vi "5GNR_Example.vi"() -> ()   [LabVIEW 2016]
uses:
  Source/SA/RFmxNR/Typedefs/NR ModAcc Configuration.ctl
  Source/SA/RFmxNR/Typedefs/NR ModAcc Results.ctl
  Source/SA/RFmxNR/Typedefs/NR ModAcc Component Carrier Results.ctl
  Source/Common/SA Common Configuration.ctl
  Source/SA/RFmxNR/Typedefs/NR Standard Configuration.ctl
  Source/SA/RFmxInstr/Typedefs/Instrument Configuration.ctl
  Source/Common/Local Oscillator Sharing Mode.ctl
  Source/Common/SA Auto Level Configuration.ctl
  Source/SA/RFmxNR/RFmxNR.lvlib
  Source/SA/RFmxInstr/RFmxInstr.lvlib
  Source/Common/Common.lvlib
panel:
  out "error out":errorcluster
  out "ModAcc Results":T1
  in  "Tab Control":enum32{"Common", "Standard", "ModAcc"}(tab)=enum."ModAcc"
  in  "Resource Name":refnum<k15>="VST"
  in  "Common Configuration":T3={"Center Frequency (Hz)"=3500000000.0, "Reference Level (dBm)"=0.0, "External Attenuation (dB)"=0.0, "Trigger Enabled"=TRUE, "Digital Trigger Source"="PXI_Trig0", "Trigger Delay (s)"=0.0, "Selected Ports"=""} {"Trigger Delay (s)" format="%.2p"; "External Attenuation (dB)" format="%.2f"; "Reference Level (dBm)" format="%.2f"; "Center Frequency (Hz)" format="%.6p"}
  in  "Instrument Configuration":T4={"LO Sharing Mode"=enum."Automatic", "Frequency Reference Source"="PXI_Clk"}
  in  "Auto Level Configuration":T6={"Enabled"=TRUE, "Measurement Interval (s)"=0.01} {"Measurement Interval (s)" min=1e-06 max=100.0 format="%.2p"}
  in  "NR Standard Configuration":T7={"Link Direction"=1, "Frequency Range"=0, "Band"=78, "Auto Resource Block Detection Enabled"=1, "Downlink Test Model"=0, "Downlink Test Model Duplex Scheme"=0, "Component Carrier Configurations"=[{"Bandwidth (Hz)"=100000000.0, "Cell ID"=0, "PUSCH Modulation Type"=1, "Subcarrier Spacing (Hz)"=30000.0, "PUSCH Resource Block Offset"=0, "PUSCH Number of Resource Blocks"=-1, "PUSCH Transform Precoding Enabled"=0, "PUSCH Slot Allocation"="0-Last", "PUSCH Symbol Allocation"="0-Last", "PUSCH DMRS Configuration Type"=0, "PUSCH Mapping Type"=0, "PUSCH DMRS Type A Position"=2, "PUSCH DMRS Duration"=1, "PUSCH DMRS Additional Positions"=0}]} {"Downlink Test Model Duplex Scheme" items=["FDD", "TDD"]; "Downlink Test Model" items=["TM1.1", "TM1.2", "TM2", "TM2a", "TM3.1", "TM3.1a", "TM3.2", "TM3.3"]; "Component Carrier Configurations"."PUSCH DMRS Additional Positions" items=["0", "1", "2", "3"]; "Component Carrier Configurations"."PUSCH DMRS Duration" items=["Single-Symbol"=1, "Double-Symbol"=2]; "Component Carrier Configurations"."PUSCH DMRS Type A Position" items=["2"=2, "3"=3]; "Component Carrier Configurations"."PUSCH Mapping Type" items=["Type A", "Type B"]; "Component Carrier Configurations"."PUSCH DMRS Configuration Type" items=["Type 1", "Type 2"]; "Component Carrier Configurations"."PUSCH Transform Precoding Enabled" items=["False", "True"]; "Component Carrier Configurations"."Subcarrier Spacing (Hz)" items=["15kHz"=15000.0, "30kHz"=30000.0, "60kHz"=60000.0, "120kHz"=120000.0]; "Component Carrier Configurations"."PUSCH Modulation Type" items=["PI/2 BPSK", "QPSK", "16 QAM", "64 QAM", "256 QAM"]; "Component Carrier Configurations"."Bandwidth (Hz)" items=["5M"=5000000.0, "10M"=10000000.0, "15M"=15000000.0, "20M"=20000000.0, "25M"=25000000.0, "30M"=30000000.0, "40M"=40000000.0, "50M"=50000000.0, "60M"=60000000.0, "70M"=70000000.0, "80M"=80000000.0, "90M"=90000000.0, "100M"=100000000.0, "200M"=200000000.0, "400M"=400000000.0]; "Auto Resource Block Detection Enabled" items=["False", "True"]; "Frequency Range" items=["Range 1", "Range 2"]; "Link Direction" items=["Downlink", "Uplink"]}
  in  "ModAcc Configuration":T8={"Measurement Length Unit"=1, "Measurement Offset"=0.0, "Measurement Length"=1.0, "EVM Unit"=0, "Averaging Enabled"=0, "Averaging Count"=10} {"Averaging Enabled" items=["False", "True"]; "EVM Unit" items=["Percentage", "dB"]; "Measurement Length Unit" items=["Slot"=1, "Subframe"=3, "Time"=6]}
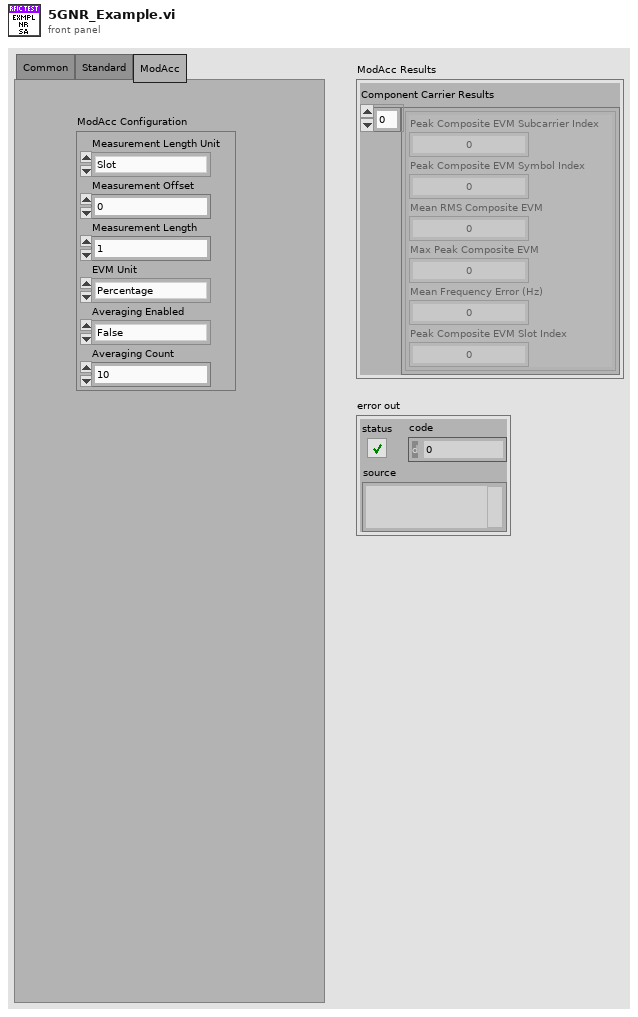
[diagram p1: front panel]
types:
  T1 = typedef "RFmxNR.lvlib/NR ModAcc Results.ctl" = cluster{"Component Carrier Results":T2[]}
  T2 = typedef "RFmxNR.lvlib/NR ModAcc Component Carrier Results.ctl" = cluster{"Peak Composite EVM Subcarrier Index":i32, "Peak Composite EVM Symbol Index":i32, "Mean RMS Composite EVM":dbl, "Max Peak Composite EVM":dbl, "Mean Frequency Error (Hz)":dbl, "Peak Composite EVM Slot Index":i32}
  T3 = typedef "Common.lvlib/SA Common Configuration.ctl" = cluster{"Center Frequency (Hz)":dbl, "Reference Level (dBm)":dbl, "External Attenuation (dB)":dbl, "Trigger Enabled":bool, "Digital Trigger Source":string, "Trigger Delay (s)":dbl, "Selected Ports":string}
  T4 = typedef "RFmxInstr.lvlib/Instrument Configuration.ctl" = cluster{"LO Sharing Mode":T5, "Frequency Reference Source":string}
  T5 = typedef "Common.lvlib/Local Oscillator Sharing Mode.ctl" = enum16{"Automatic", "None"}
  T6 = typedef "Common.lvlib/SA Auto Level Configuration.ctl" = cluster{"Enabled":bool, "Measurement Interval (s)":dbl}
  T7 = typedef "RFmxNR.lvlib/NR Standard Configuration.ctl" = cluster{"Link Direction":i32, "Frequency Range":i32, "Band":i32, "Auto Resource Block Detection Enabled":i32, "Downlink Test Model":i32, "Downlink Test Model Duplex Scheme":i32, "Component Carrier Configurations":cluster{"Bandwidth (Hz)":dbl, "Cell ID":i32, "PUSCH Modulation Type":i32, "Subcarrier Spacing (Hz)":dbl, "PUSCH Resource Block Offset":i32, "PUSCH Number of Resource Blocks":i32, "PUSCH Transform Precoding Enabled":i32, "PUSCH Slot Allocation":string, "PUSCH Symbol Allocation":string, "PUSCH DMRS Configuration Type":i32, "PUSCH Mapping Type":i32, "PUSCH DMRS Type A Position":i32, "PUSCH DMRS Duration":i32, "PUSCH DMRS Additional Positions":i32}[]}
  T8 = typedef "RFmxNR.lvlib/NR ModAcc Configuration.ctl" = cluster{"Measurement Length Unit":i32, "Measurement Offset":dbl, "Measurement Length":dbl, "EVM Unit":i32, "Averaging Enabled":i32, "Averaging Count":i32}
  T9 = enum16{"ModAcc", "SEM", "ACP", "CHP", "OBW", "PVT"}[]
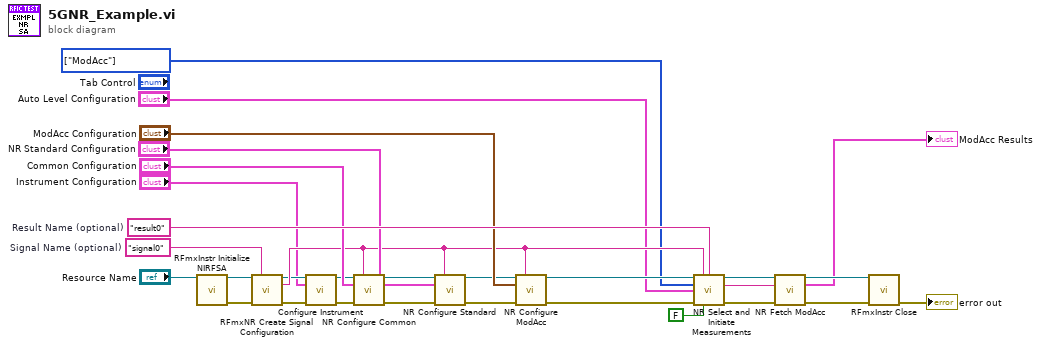
[diagram p0: block diagram]
diagram:
  w3 = T9 [enum."ModAcc"] items=["ModAcc", "SEM", "ACP", "CHP", "OBW", "PVT"] ("Measurements")
  w19 = "result0"  # Result Name (optional)
  w20 = "signal0"  # Signal Name (optional)
  n1 = call <vilib>:"RFmxInstr Initialize NIRFSA.vi"("Resource Name"="Resource Name") -> ("Instrument Handle Out"=w21:refnum<k21>, "error out"=w30:errorcluster)  [unwired: 12 in, 1 out]
  n2 = call <vilib>:"RFmxNR Create Signal Configuration.vi"("Instrument Handle In"=w21, "Signal Name"=w20, "error in (no error)"=w30) -> ("Instrument Handle Out"=w8:refnum<k21>, "Selector String Out"=w9:string, "error out"=w6:errorcluster)  [unwired: 10 in]
  n3 = call "Configure Instrument.vi"("Instrument Handle In"=w8, "Instrument Configuration"="Instrument Configuration", "error in (no error)"=w6) -> ("Instrument Handle Out"=w7:refnum<k21>, "error out"=w5:errorcluster)  [unwired: 11 in]
  n4 = call "NR Configure Common.vi"("RFmx Handle In"=w7, "Selector String"=w9, "Common Configuration"="Common Configuration", "error in (no error)"=w5) -> ("RFmx Handle Out"=w14:refnum<k21>, "error out"=w11:errorcluster)  [unwired: 10 in]
  n5 = call "NR Configure Standard.vi"("RFmx Handle In"=w14, "Selector String"=w9, "NR Standard Configuration"="NR Standard Configuration", "error in (no error)"=w11) -> ("RFmx Handle Out"=w13:refnum<k21>, "error out"=w12:errorcluster)  [unwired: 10 in]
  n6 = call "NR Configure ModAcc.vi"("RFmx Handle In"=w13, "Selector String"=w9, "NR ModAcc Configuration"="ModAcc Configuration", "error in (no error)"=w12) -> ("RFmx Handle Out"=w28:refnum<k21>, "error out"=w27:errorcluster)  [unwired: 10 in]
  n7 = call "NR Select and Initiate Measurements.vi"("Instrument Handle In"=w28, "Selector String"=w9, "Result Name"=w19, "Measurements"=w3, "Auto Level Configuration"="Auto Level Configuration", "error in (no error)"=w27, "Enable All Traces (F)"=FALSE) -> ("Instrument Handle Out"=w26:refnum<k21>, "Selector String Out"=w16:string, "error out"=w25:errorcluster)  [unwired: 6 in]
  n8 = call "NR Fetch ModAcc.vi"("RFmx Handle In"=w26, "Selector String"=w16, "error in (no error)"=w25) -> ("RFmx Handle Out"=w24:refnum<k21>, "ModAcc Results"=→"ModAcc Results":T1, "error out"=w18:errorcluster)  [unwired: 10 in]
  n9 = call <vilib>:"RFmxInstr Close.vi"("Instrument Handle In"=w24, "error in (no error)"=w18) -> ("error out"=→"error out":errorcluster)  [unwired: 13 in]
